vi "CompileActionSettings.vi"(8 "error in (no error)":errorcluster, 11 "Item Ref in":T1 format="%.0x") -> (0 "error out":errorcluster, 2 "Item Ref out":T1 format="%.0x", 3 "Action Settings":T2)   [LabVIEW 2024, in "Embedded TDMS Logger System Explorer.lvlib"]
uses:
  Embedded TDMS Logger System Explorer.lvlib
  <vilib>/NI VeriStand/Custom Device API/Custom Device API.lvlib
  <vilib>/NI VeriStand/Custom Device API/Get Item Property (Boolean).vi
  <vilib>/NI VeriStand/Custom Device API/Get Item Property (String).vi
  <vilib>/NI VeriStand/Custom Device API/Custom Device Item Ref.ctl
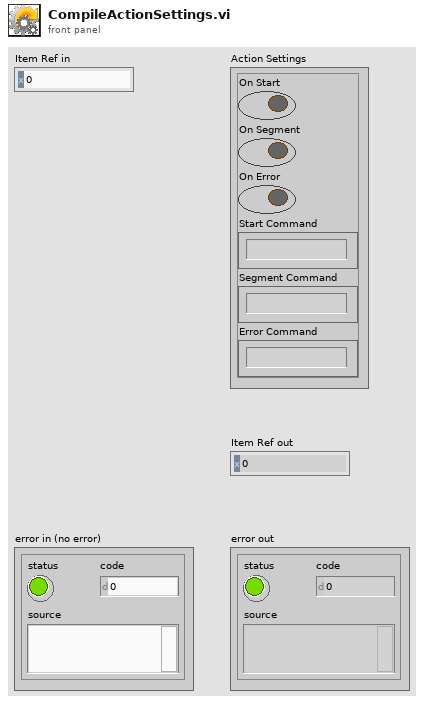
[diagram p1: front panel]
types:
  T1 = typedef "Custom Device API.lvlib/Custom Device Item Ref.ctl" = u64
  T2 = cluster{"On Start":bool, "On Segment":bool, "On Error":bool, "Start Command":string, "Segment Command":string, "Error Command":string}
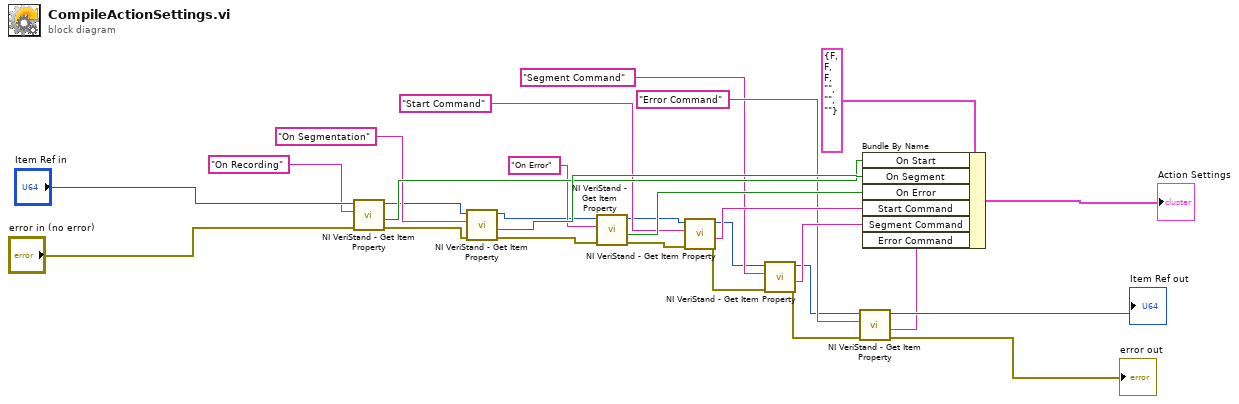
[diagram p0: block diagram]
diagram:
  n1 = call-poly <vilib>:"NI VeriStand - Get Item Property.vi"("error in (no error)"="error in (no error)", "Property Name"="On Recording", "Item Ref in"="Item Ref in") -> ("error out"=w8:errorcluster, "Value"=w23:bool, "Item Ref out"=w3:T1)  [unwired: 5 in, 1 out]
  n2 = call-poly <vilib>:"NI VeriStand - Get Item Property.vi"("error in (no error)"=w8, "Property Name"="On Segmentation", "Item Ref in"=w3) -> ("error out"=w10:errorcluster, "Value"=w24:bool, "Item Ref out"=w2:T1)  [unwired: 5 in, 1 out]
  n3 = call-poly <vilib>:"NI VeriStand - Get Item Property.vi"("error in (no error)"=w10, "Property Name"="On Error", "Item Ref in"=w2) -> ("error out"=w12:errorcluster, "Value"=w25:bool, "Item Ref out"=w11:T1)  [unwired: 5 in, 1 out]
  n4 = call-poly <vilib>:"NI VeriStand - Get Item Property.vi"("error in (no error)"=w12, "Property Name"="Start Command", "Item Ref in"=w11) -> ("error out"=w15:errorcluster, "Value"=w20:string, "Item Ref out"=w14:T1)  [unwired: 5 in, 1 out]
  n5 = call-poly <vilib>:"NI VeriStand - Get Item Property.vi"("error in (no error)"=w15, "Property Name"="Segment Command", "Item Ref in"=w14) -> ("error out"=w16:errorcluster, "Value"=w21:string, "Item Ref out"=w13:T1)  [unwired: 5 in, 1 out]
  n6 = call-poly <vilib>:"NI VeriStand - Get Item Property.vi"("error in (no error)"=w16, "Property Name"="Error Command", "Item Ref in"=w13) -> ("error out"=→"error out":errorcluster, "Value"=w22:string, "Item Ref out"=→"Item Ref out":T1)  [unwired: 5 in, 1 out]
  n7 = Bundle By Name(cluster=T2 {"On Start"=FALSE, "On Segment"=FALSE, "On Error"=FALSE, "Start Command"="", "Segment Command"="", "Error Command"=""} ("Action Settings"), "On Start"=w23, "On Segment"=w24, "On Error"=w25, "Start Command"=w20, "Segment Command"=w21, "Error Command"=w22) -> (→"Action Settings":T2)
